vi "Write to Log File.vi"(8 "error in (no error)":errorcluster, 10 "Array of Waveforms":waveform(dbl)[](array[waveform]), 11 "Log File in":refnum<k34>) -> (0 "error out":errorcluster)   [LabVIEW 2017, in "Logging.lvlib"]
uses:
  Logging.lvlib
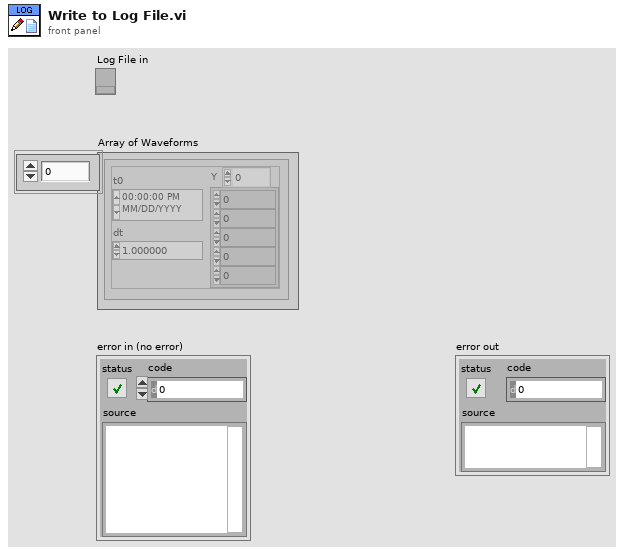
[diagram p1: front panel]
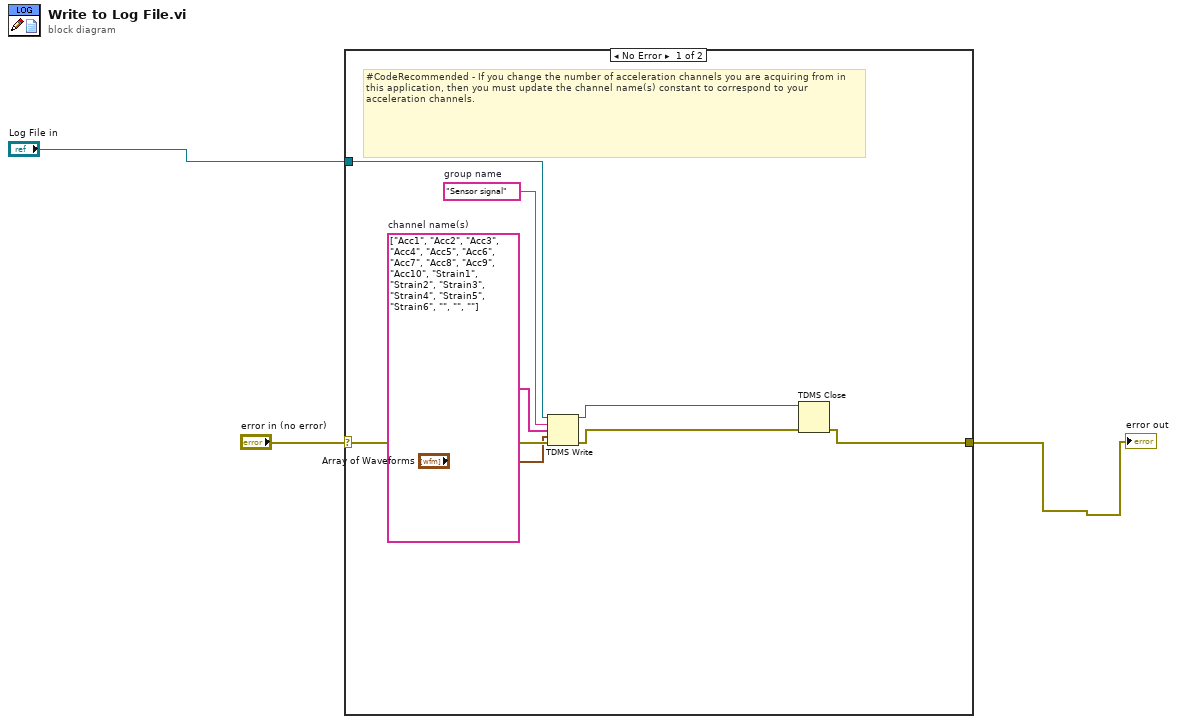
[diagram p0: block diagram]
diagram:
  n1 = case shown="No Error" "error in (no error)" {
    selector: "error in (no error)" -> [w9 w12]
    tunnel: "Log File in" -> [w10 _]
    tunnel: [w4 w12] -> w1
    frame No Error {
      w8 = string[] ["Acc1", "Acc2", "Acc3", "Acc4", "Acc5", "Acc6", "Acc7", "Acc8", "Acc9", "Acc10", "Strain1", "Strain2", "Strain3", "Strain4", "Strain5", "Strain6", "", "", ""]  # channel name(s)
      w11 = "Sensor signal"  # group name
      # "#CodeRecommended - If you change the number of acceleration channels you are acquiring from in this application, then you must update the channel name(s) constant to correspond to your acceleration channels."
      n2 = TDMS Write(0:w10, 5:w11, 7:w8, 9:"Array of Waveforms", 11:w9) -> (4:w6:refnum<k34>, 15:w5:errorcluster)  [unwired: 1 in, 2 out]
      n3 = TDMS Close(8:w5, 11:w6) -> (0:w4:errorcluster)  [unwired: 1 out]
    }
    frame Error {
    }
  }
  "error out" <- w1
